vi "Sign Out.vi"(0 "ICanCommunicate In":refnum<class "Process.lvclass">, 7 "Message Handler":refnum<class "ICanCommunicate.lvclass">, 11 "Error In":errorcluster) -> (4 "ICanCommunicate Out":refnum<class "Process.lvclass">, 15 "Error Out":errorcluster)   [LabVIEW 2023, in "Process.lvclass"]
uses:
  Process.lvclass
  Interfaces/ICanCommunicate/ICanCommunicate.lvclass
  Subclasses/Message Handler/Message Handler.lvclass
  Process.lvclass/Process.ctl
  H:/Desktop/LabVIEW/LabView Repo/Framework/Classes/Processes/Process/Process.lvclass
  H:/Desktop/LabVIEW/LabView Repo/Framework/Interfaces/ICanCommunicate/ICanCommunicate.lvclass
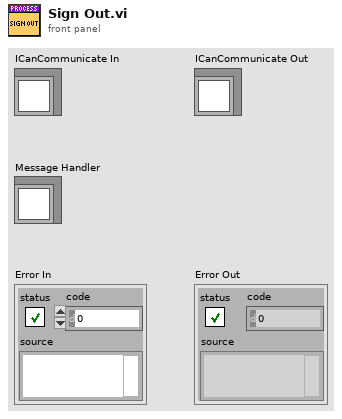
[diagram p1: front panel]
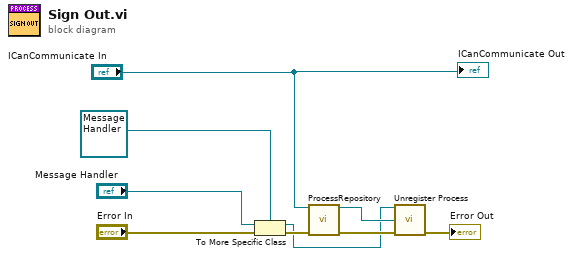
[diagram p0: block diagram]
diagram:
  n1 = To More Specific Class(target class=refnum<class "Message Handler.lvclass"> refnum ("Process"), reference="Message Handler", error in="Error In") -> (specific class reference=w6:refnum<class "Message Handler.lvclass">, error out=w7:errorcluster)
  n2 = call-dynamic "ProcessRepository.vi"("Process In"="ICanCommunicate In", "Error In"=w7) -> ("Process Out"=w9:refnum<class "Process.lvclass">, "Error Out"=w8:errorcluster)  [unwired: 7 in, 5 out]
  n3 = call-dynamic "Unregister Process.vi"("Message Handler In"=w6, "Process"=w9, "Error In"=w8) -> ("Error Out"=→"Error Out":errorcluster)  [unwired: 11 in, 1 out]
  "ICanCommunicate Out" <- "ICanCommunicate In"
